vi "LabVIEW Build UI.vi"() -> ()   [LabVIEW 2014, in "LabVIEW Build Node.lvclass"]
uses:
  LabVIEW Build Node.lvclass
  <vilib>/ni/Configuration Framework/Node/NodeRef.ctl
  <vilib>/ni/Configuration Framework/Node/NISE_CEF_Node.lvclass
  <vilib>/ni/AMC/Message Queue.ctl
  <vilib>/ni/AMC/Message.ctl
  <vilib>/ni/Tools/Keyed Array/KeyedArray.ctl
  <vilib>/ni/Configuration Framework/Node/UserEventRef.ctl
  <vilib>/ni/Configuration Framework/Controls/EventCluster.ctl
  LabVIEW Build Node.lvclass/LabVIEW Build Node.ctl
  Classes/Build Job/Build Job.lvclass/Build Job.ctl
  <vilib>/ni/AMC/Create Single Message.vi
  <vilib>/ni/AMC/Update Message Routing Info.vi
  <vilib>/ni/AMC/Send Message.vi
  <vilib>/ni/AMC/AMC.lvlib
  CI Project Builder.lvlib
  Classes/Build Job/Build Job.lvclass
  <vilib>/ni/Tools/Keyed Array/Tools_KeyedArray.lvlib
  <vilib>/ni/Configuration Framework/NISE_CEF_TreeControl.lvlib
panel:
  in  "Target":string(combo)
  in  "Build Spec":string(combo) caption="Build Specification"
  in  "Description":string="brandyn.adderley@ni.com"
  in  "Project Path":path=path "C:/Projects/LabVIEW Continuous Integration/LabVIEW Continuous Integration.lvproj"
  in  "Increment":bool caption="Increment Version Automatically?"
  in  "user event":T1
  in  "main queue":T2
  in  "node ref":T3
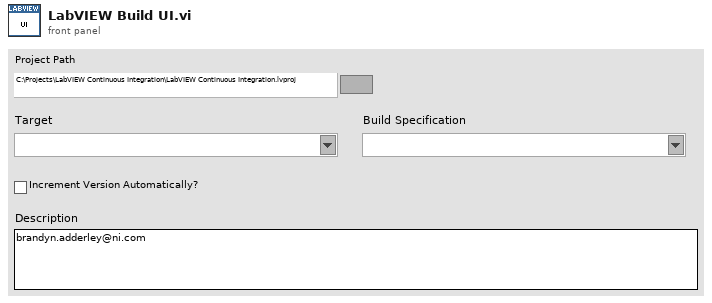
[diagram p1: front panel]
types:
  T1 = typedef "NISE_CEF_Node.lvclass/UserEventRef.ctl" = refnum<user-event>
  T2 = typedef "AMC.lvlib/Message Queue.ctl" = refnum<queue>
  T3 = typedef "NISE_CEF_Node.lvclass/NodeRef.ctl" = refnum<data-value>
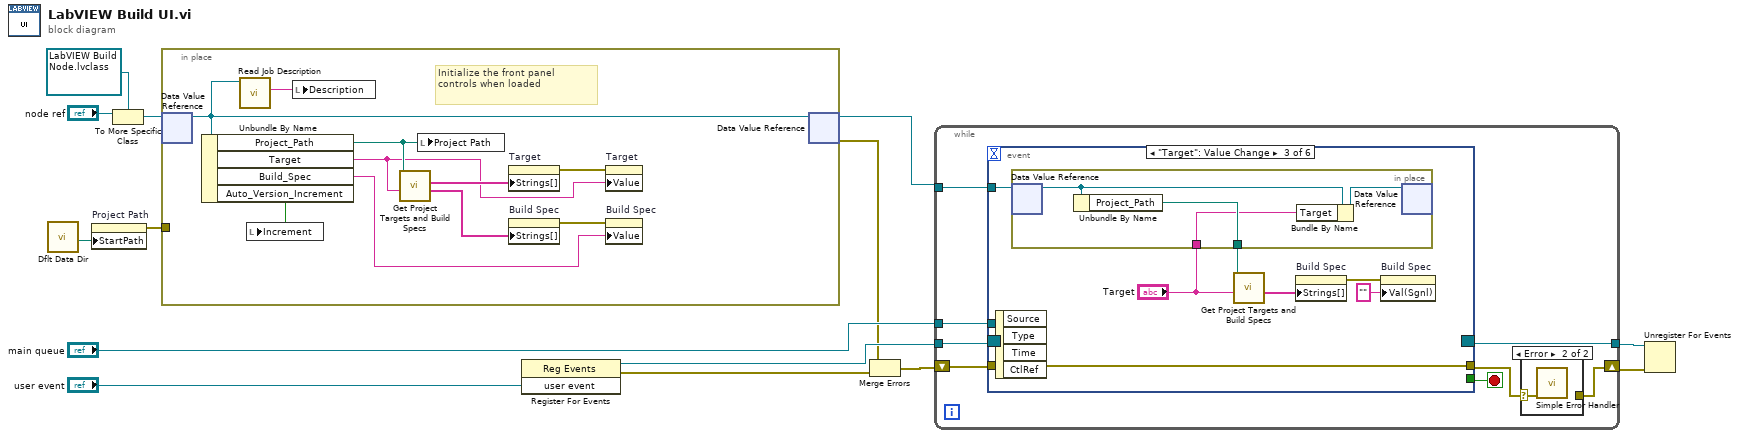
[diagram p0: block diagram]
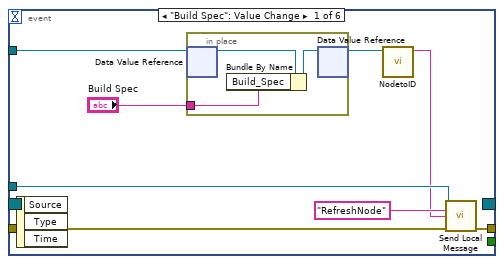
[diagram p3: hidden frame]
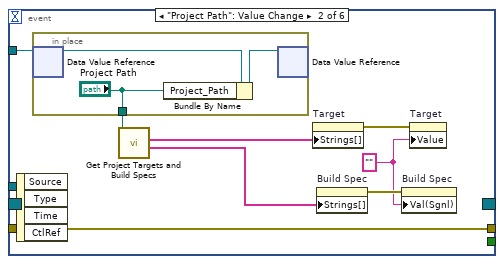
[diagram p4: hidden frame]
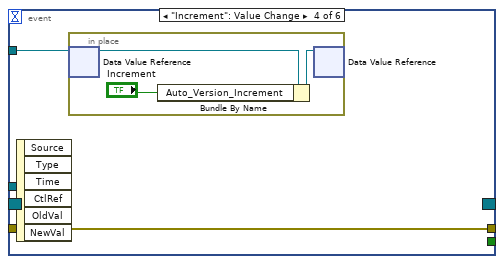
[diagram p5: hidden frame]
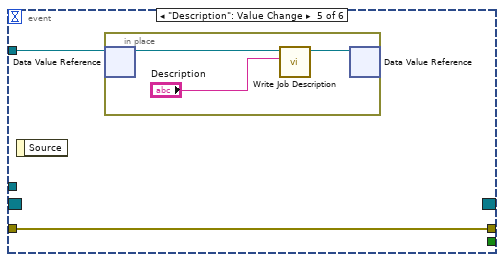
[diagram p6: hidden frame]
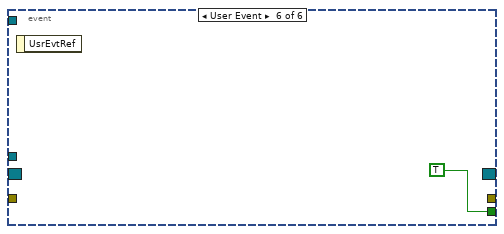
[diagram p7: hidden frame]
diagram:
  n1 = call <vilib>:"Dflt Data Dir.vi"() -> ("App:Default Data Directory"=w2:path)
  n2 = property on="Project Path" class="Path"("StartPath"=w2) -> (error out=w1:errorcluster)  [unwired: 2 in, 1 out]
  n3 = To More Specific Class(target class=refnum<data-value> refnum ("data value reference"), reference="node ref") -> (specific class reference=w8:refnum<data-value>)  [unwired: 1 in, 1 out]
  n4 = in-place {
    in-place-border: w1 -> [_]
    # "Initialize the front panel controls when loaded"
    n5 = in-place-dvr #1(w8) -> (w21:refnum<class "LabVIEW Build Node.lvclass">)  [unwired: 1 out]
    n6 = Unbundle By Name(w21) -> ("Project_Path"=w23:path, "Target"=w15:string, "Build_Spec"=w19:string, "Auto_Version_Increment"=w24:bool)
    n7 = call-dynamic "Read Job Description.vi"("Build Job in"=w21) -> ("Job Description"=w20:string)  [unwired: 10 in]
    n8 = local write "Increment"(w24) -> ()
    n9 = local write "Description"(w20) -> ()
    n10 = call "Get Project Targets and Build Specs.vi"("Name of target (My Computer)"=w15, "Path to project"=w23) -> ("Build Specs"=w18:string[], "All Targets"=w17:string[])  [unwired: 7 in, 1 out]
    n11 = local write "Project Path"(w23) -> ()
    n12 = property on="Target" class="CmbBox"("Strings[]"=w17) -> (error out=w16:errorcluster)  [unwired: 2 in, 1 out]
    n13 = property on="Build Spec" class="CmbBox"("Strings[]"=w18) -> (error out=w22:errorcluster)  [unwired: 2 in, 1 out]
    n14 = property on="Target" class="CmbBox"(error in=w16, "Value"=w15) -> ()  [unwired: 1 in, 2 out]
    n15 = property on="Build Spec" class="CmbBox"(error in=w22, "Value"=w19) -> ()  [unwired: 1 in, 2 out]
    n16 = in-place-dvr #1(w21) -> (w3:refnum<data-value>, w5:errorcluster)
  }
  n17 = register-events("user event") -> (reference out=w12:refnum<event-registration>, error out=w6:errorcluster)  [unwired: 2 in]
  n18 = Merge Errors(w5, w6) -> (w4:errorcluster)
  n19 = while {
    tunnel: w3 -> [w32]
    tunnel: "main queue" -> [w31]
    tunnel: w12 -> [w30]
    tunnel: [w29] -> w11
    shift-right: [w25] -> w10
    shift-left: w4 -> [w28]
    stop <- w27 stop-if-true
    n20 = event shown="[2] \"Target\": Value Change" {
      selector: w30 -> [_ _ _ _ _ _]
      dyn-events: [_ _ _ _ _ _] -> w29
      timeout: _ -> [_ _ _ _ _ _]
      tunnel: w32 -> [w40 w53 w63 w69 w74 _]
      tunnel: w31 -> [w41 _ _ _ _ _]
      tunnel: [_ _ _ _ _ TRUE] -> w27
      tunnel: [w38 w52 w62 w68 w73 _] -> w26
      tunnel: w28 -> [w37 w52 w62 w68 w73 _]
      event "Build Spec": Value Change {
        n21 = event-data() -> ()  [unwired: 1 in, 3 out]
        n22 = in-place {
          in-place-border: "Build Spec" -> [w43]
          n23 = in-place-dvr #2(w40) -> (w45:refnum<class "LabVIEW Build Node.lvclass">)  [unwired: 1 out]
          n24 = Bundle By Name(cluster=w45, "Build_Spec"=w43) -> (w44:refnum<class "LabVIEW Build Node.lvclass">)
          n25 = in-place-dvr #2(w44) -> (w36:refnum<data-value>)  [unwired: 1 out]
        }
        n26 = call <vilib>:"NodetoID.vi"("node ref"=w36) -> ("ID"=w39:string)  [unwired: 9 in, 1 out]
        n27 = call <vilib>:"Send Local Message.vi"("message queue in"=w41, "message name"="RefreshNode" ("Message Name"), "message value"=w39, "error in"=w37) -> ("error out"=w38:errorcluster)  [unwired: 9 in, 2 out]
      }
      event "Project Path": Value Change {
        w46 = "" ("Value (Signaling)")
        n28 = event-data() -> ()  [unwired: 1 in, 4 out]
        n29 = in-place {
          in-place-border: ["Project Path"] -> w50
          n30 = in-place-dvr #3(w53) -> (w56:refnum<class "LabVIEW Build Node.lvclass">)  [unwired: 1 out]
          n31 = Bundle By Name(cluster=w56, "Project_Path"="Project Path") -> (w55:refnum<class "LabVIEW Build Node.lvclass">)
          n32 = in-place-dvr #3(w55) -> ()  [unwired: 2 out]
        }
        n33 = call "Get Project Targets and Build Specs.vi"("Path to project"=w50) -> ("Build Specs"=w49:string[], "All Targets"=w47:string[])  [unwired: 8 in, 1 out]
        n34 = property on="Target" class="CmbBox"("Strings[]"=w47) -> (error out=w48:errorcluster)  [unwired: 2 in, 1 out]
        n35 = property on="Build Spec" class="CmbBox"("Strings[]"=w49) -> (error out=w51:errorcluster)  [unwired: 2 in, 1 out]
        n36 = property on="Build Spec" class="CmbBox"(error in=w51, "Val(Sgnl)"=w46) -> ()  [unwired: 1 in, 2 out]
        n37 = property on="Target" class="CmbBox"(error in=w48, "Value"=w46) -> ()  [unwired: 1 in, 2 out]
      }
      event "Target": Value Change {
        n38 = event-data() -> ()  [unwired: 1 in, 4 out]
        n39 = in-place {
          in-place-border: [w65] -> w60
          in-place-border: "Target" -> [w64]
          n40 = in-place-dvr #4(w63) -> (w66:refnum<class "LabVIEW Build Node.lvclass">)  [unwired: 1 out]
          n41 = Unbundle By Name(w66) -> ("Project_Path"=w65:path)
          n42 = Bundle By Name(cluster=w66, "Target"=w64) -> (w67:refnum<class "LabVIEW Build Node.lvclass">)
          n43 = in-place-dvr #4(w67) -> ()  [unwired: 2 out]
        }
        n44 = call "Get Project Targets and Build Specs.vi"("Name of target (My Computer)"="Target", "Path to project"=w60) -> ("Build Specs"=w59:string[])  [unwired: 7 in, 2 out]
        n45 = property on="Build Spec" class="CmbBox"("Strings[]"=w59) -> (error out=w61:errorcluster)  [unwired: 2 in, 1 out]
        n46 = property on="Build Spec" class="CmbBox"(error in=w61, "Val(Sgnl)"="" ("Value (Signaling)")) -> ()  [unwired: 1 in, 2 out]
      }
      event "Increment": Value Change {
        n47 = event-data() -> ()  [unwired: 1 in, 6 out]
        n48 = in-place {
          n49 = in-place-dvr #5(w69) -> (w72:refnum<class "LabVIEW Build Node.lvclass">)  [unwired: 1 out]
          n50 = Bundle By Name(cluster=w72, "Auto_Version_Increment"="Increment") -> (w71:refnum<class "LabVIEW Build Node.lvclass">)
          n51 = in-place-dvr #5(w71) -> ()  [unwired: 2 out]
        }
      }
      event "Description": Value Change {
        n52 = event-data() -> ()  [unwired: 1 in, 1 out]
        n53 = in-place {
          n54 = in-place-dvr #6(w74) -> (w77:refnum<class "LabVIEW Build Node.lvclass">)  [unwired: 1 out]
          n55 = call "Write Job Description.vi"("Job Description"="Description", "Build Job in"=w77) -> ("Build Job out"=w76:refnum<class "LabVIEW Build Node.lvclass">)  [unwired: 9 in]
          n56 = in-place-dvr #6(w76) -> ()  [unwired: 2 out]
        }
      }
      event User Event {
        n57 = event-data() -> ()  [unwired: 1 in, 1 out]
      }
    }
    n58 = case shown="Error" w26 {
      selector: w26 -> [w33 w34]
      tunnel: [w33 _] -> w25
      frame No Error {
      }
      frame Error {
        n59 = call <vilib>:"Simple Error Handler.vi"("error in (no error)"=w34) -> ()  [unwired: 4 in, 5 out]
      }
    }
  }
  n60 = Unregister For Events(event registration refnum=w11, error in=w10) -> ()  [unwired: 1 out]
